vi "GenericSweep - Multiple sweeps.vi"() -> ()   [LabVIEW 2017]
doc: "This example performs multiple generic sweeps with different limits.\n\n- Nanonis Programming Interface -"
uses:
  Nanonis Prog Interface.lvlib
panel:
  out "XY Graph":cluster{"Data":sgl[], "Data":sgl[]}(graph)
  # "Example for the Nanonis SPM Control software programming interface (see diagram)"
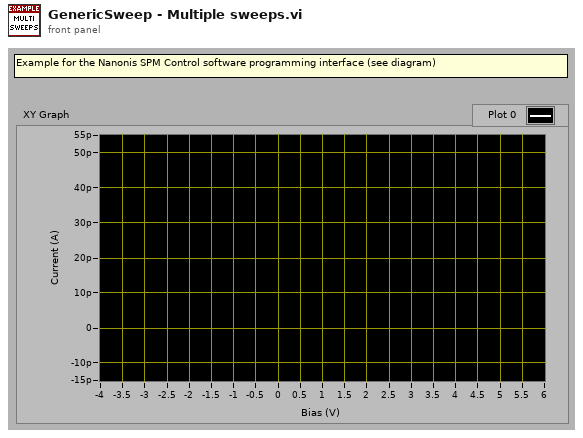
[diagram p1: front panel]
types:
  T1 = enum16{"no change", "turn off", "don't turn off"}
  T2 = cluster{"Initial Settling time (ms) (NaN=no change)":sgl, "Settling time (ms) (NaN=no change)":sgl, "Period (ms) (0=no change)":u16}
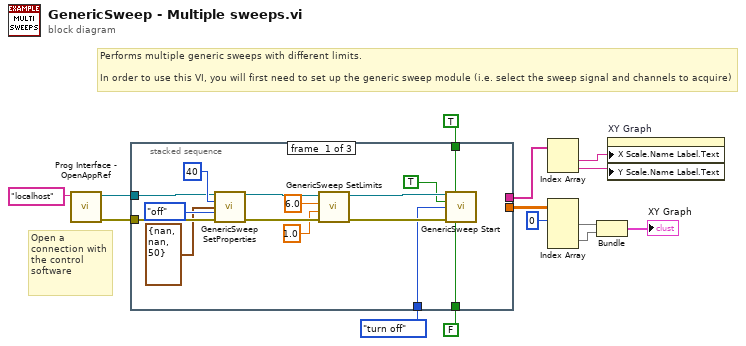
[diagram p0: block diagram]
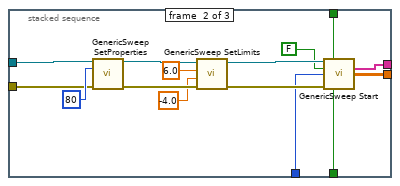
[diagram p2: hidden frame]
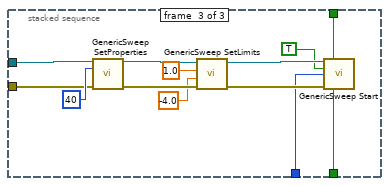
[diagram p3: hidden frame]
diagram:
  # "Open a connection with the control\nsoftware"
  # "Performs multiple generic sweeps with different limits.\n\nIn order to use this VI, you will first need to set up the generic sweep module (i.e. select the sweep signal and channels to acquire)"
  n1 = call <userlib>:"Prog Interface - OpenAppRef.vi"("Machine name (local machine IP)"="localhost" ("Machine name (localhost)")) -> ("Error out"=w3:errorcluster, "Application reference"=w1:refnum<vi>)  [unwired: 5 in]
  n2 = stacked-sequence {
    tunnel: [_ w40 _] -> w14
    tunnel: [_ w39 _] -> w9
    tunnel: T1."turn off" ("Z-Controller (no change)") -> [w16 w31 w46]
    tunnel: FALSE ("Reset Signal? (T)") -> [w24 w38 w53]
    tunnel: TRUE ("Get Data (F)") -> [w23 w37 w52]
    tunnel: w3 -> [w22 w36 w51]
    tunnel: w1 -> [w21 w30 w45]
    frame #0 {
      n3 = call <userlib>:"GenericSweep SetProperties.vi"("Application ref in"=w21, "Number of steps (0=no change)"=u16 40 ("Number of Steps\n(0=no change)"), "Times (ms)"=T2 {"Initial Settling time (ms) (NaN=no change)"=nan, "Settling time (ms) (NaN=no change)"=nan, "Period (ms) (0=no change)"=50}, "Autosave (no change)"=enum16{"no change", "on", "off"}."off" ("Autosave"), "error in (no error)"=w22) -> ("Application ref out"=w19:refnum<vi>, "error out"=w27:errorcluster)  [unwired: 9 in]
      n4 = call <userlib>:"GenericSweep SetLimits.vi"("error in (no error)"=w27, "Lower limit"=sgl 1.0 ("Lower Limit"), "Upper limit"=sgl 6.0 ("Upper Limit"), "Application ref in"=w19) -> ("error out"=w25:errorcluster, "Application ref out"=w18:refnum<vi>)  [unwired: 4 in]
      n5 = call <userlib>:"GenericSweep Start.vi"("Application ref in"=w18, "Get data (F)"=w23, "Sweep dir (T = up)"=TRUE, "Z-Controller (no change)"=w16, "error in (no error)"=w25, "Reset signal (T)"=w24) -> ()  [unwired: 6 in, 4 out]
    }
    frame #1 {
      n6 = call <userlib>:"GenericSweep SetProperties.vi"("Application ref in"=w30, "Number of steps (0=no change)"=u16 80 ("Number of Steps\n(0=no change)"), "error in (no error)"=w36) -> ("Application ref out"=w34:refnum<vi>, "error out"=w43:errorcluster)  [unwired: 11 in]
      n7 = call <userlib>:"GenericSweep SetLimits.vi"("error in (no error)"=w43, "Lower limit"=sgl -4.0 ("Lower Limit"), "Upper limit"=sgl 6.0 ("Upper Limit"), "Application ref in"=w34) -> ("error out"=w41:errorcluster, "Application ref out"=w33:refnum<vi>)  [unwired: 4 in]
      n8 = call <userlib>:"GenericSweep Start.vi"("Application ref in"=w33, "Get data (F)"=w37, "Sweep dir (T = up)"=FALSE, "Z-Controller (no change)"=w31, "error in (no error)"=w41, "Reset signal (T)"=w38) -> ("Channels"=w39:string[], "Data"=w40:sgl[][])  [unwired: 6 in, 2 out]
    }
    frame #2 {
      n9 = call <userlib>:"GenericSweep SetProperties.vi"("Application ref in"=w45, "Number of steps (0=no change)"=u16 40 ("Number of Steps\n(0=no change)"), "error in (no error)"=w51) -> ("Application ref out"=w49:refnum<vi>, "error out"=w56:errorcluster)  [unwired: 11 in]
      n10 = call <userlib>:"GenericSweep SetLimits.vi"("error in (no error)"=w56, "Lower limit"=sgl -4.0 ("Lower Limit"), "Upper limit"=sgl 1.0 ("Upper Limit"), "Application ref in"=w49) -> ("error out"=w54:errorcluster, "Application ref out"=w48:refnum<vi>)  [unwired: 4 in]
      n11 = call <userlib>:"GenericSweep Start.vi"("Application ref in"=w48, "Get data (F)"=w52, "Sweep dir (T = up)"=TRUE, "Z-Controller (no change)"=w46, "error in (no error)"=w54, "Reset signal (T)"=w53) -> ()  [unwired: 6 in, 4 out]
    }
  }
  n12 = Index Array(array=w9) -> (element #1=w8:string, element #2=w7:string)  [unwired: 2 in]
  n13 = Index Array(array=w14, index (row) #1=0 ("index (row)")) -> (element #1=w12:sgl[], element #2=w11:sgl[])  [unwired: 3 in]
  n14 = Bundle("Data"=w12, "Data"=w11) -> (→"XY Graph":cluster{"Data":sgl[], "Data":sgl[]})  [unwired: 1 in]
  n15 = property on="XY Graph" class="XYGraph (strict)"("X Scale.Name Label.Text"=w8, "Y Scale.Name Label.Text"=w7) -> ()  [unwired: 2 in, 2 out]
